vi "Find DO Tags.vi"(8 "error in (no error)":errorcluster, 11 "DAQ State in":T1) -> (0 "error out":errorcluster, 2 "Task D-O Channels":string[][](array[string]), 3 "DAQ State out":T1)   [LabVIEW 2018, in "DAQ.lvlib"]
uses:
  DAQ/DAQ.lvlib
  Hardware Configuration.ctl
  Task Cluster.ctl
  <resource>/objmgr/daqmx.rc
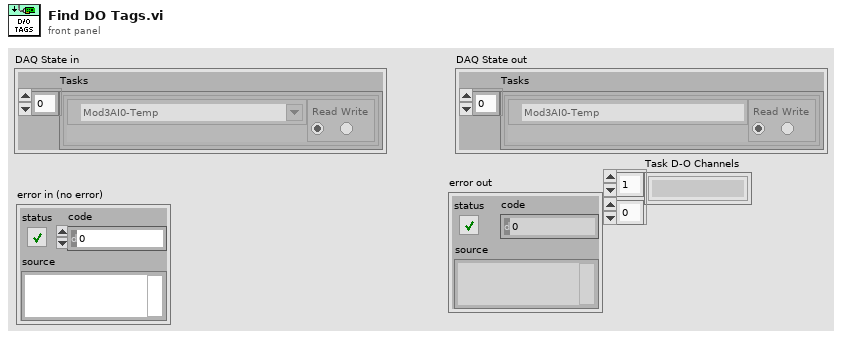
[diagram p1: front panel]
types:
  T1 = typedef "DAQ.lvlib/Hardware Configuration.ctl" = cluster{"Tasks":T2[]}
  T2 = typedef "Task Cluster.ctl" = cluster{"DAQmx Task":refnum<k21>, "Read-Write Radio":enum32{"Read", "Write"}}
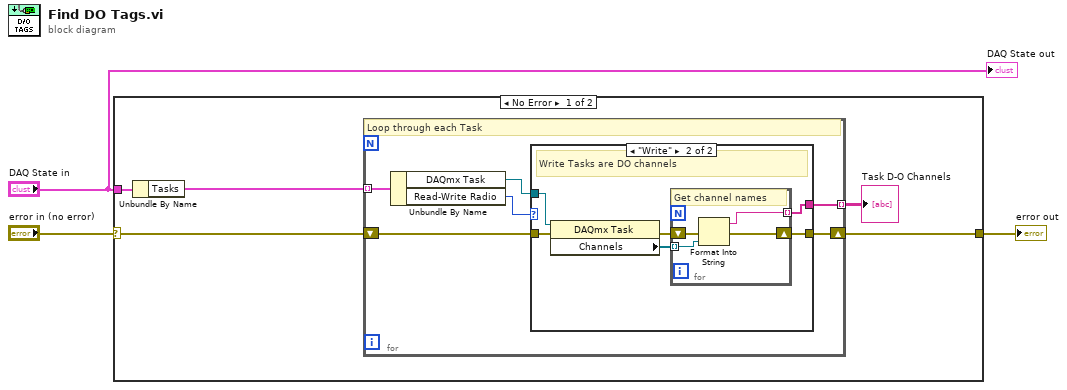
[diagram p0: block diagram]
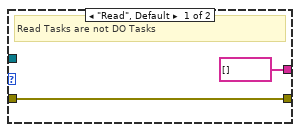
[diagram p2: hidden frame]
diagram:
  n1 = case shown="No Error" "error in (no error)" {
    selector: "error in (no error)" -> [w4 w27]
    tunnel: "DAQ State in" -> [w7 _]
    tunnel: [w6 w27] -> w1
    frame No Error {
      n2 = Unbundle By Name(w7) -> ("Tasks"=w8:T2[])
      n3 = for {
        tunnel: w8 -> [w14] mode=indexing
        shift-right: [w11] -> w6
        shift-left: w4 -> [w9]
        tunnel: [w12] -> w5 mode=indexing
        # "Loop through each Task"
        n4 = Unbundle By Name(w14) -> ("DAQmx Task"=w10:refnum<k21>, "Read-Write Radio"=w13:enum32{"Read", "Write"})
        n5 = case shown="\"Write\"" w13 {
          tunnel: [string[] [] w17] -> w12
          tunnel: [w16 w22] -> w11
          tunnel: w10 -> [_ w21]
          tunnel: w9 -> [w16 w20]
          frame "Read", Default {
            # "Read Tasks are not DO Tasks"
          }
          frame "Write" {
            # "Write Tasks are DO channels"
            n6 = property class="DAQmx Task"(reference=w21, error in=w20) -> (error out=w19:errorcluster, "Channels"=w18:refnum<k21>[])  [unwired: 1 out]
            n7 = for {
              tunnel: w18 -> [w26] mode=indexing
              shift-right: [w23] -> w22
              shift-left: w19 -> [w25]
              tunnel: [w24] -> w17 mode=indexing
              # "Get channel names"
              n8 = Format Into String(error in=w25, w26) -> (resulting string=w24:string, error out=w23:errorcluster)  [unwired: 2 in]
            }
          }
        }
      }
      "Task D-O Channels" <- w5
    }
    frame Error {
    }
  }
  "error out" <- w1
  "DAQ State out" <- "DAQ State in"
